vi "Log Into File.vi"(8 "error in":errorcluster, 10 "Memory Information":dbl[](array[numeric]), 11 "file path in":path) -> (0 "error out":errorcluster, 3 "file path out":path)   [LabVIEW 2016]
uses:
  <vilib>/Utility/file.llb/Write Delimited Spreadsheet (string).vi
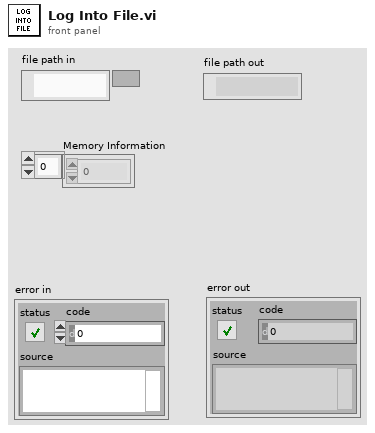
[diagram p1: front panel]
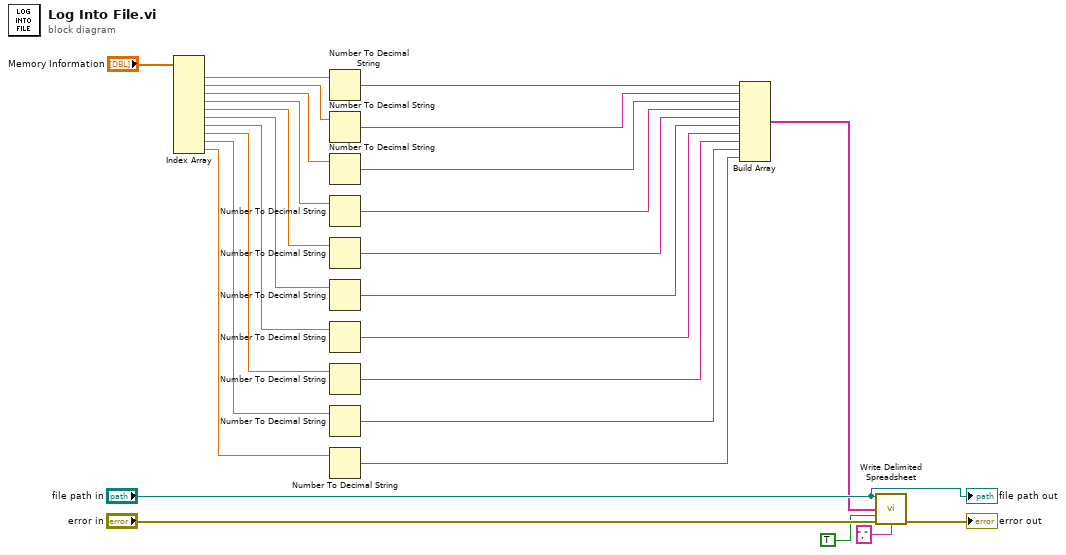
[diagram p0: block diagram]
diagram:
  n1 = Index Array(array="Memory Information") -> (element #1=w26:dbl, element #2=w21:dbl, element #3=w20:dbl, element #4=w19:dbl, element #5=w18:dbl, element #6=w17:dbl, element #7=w16:dbl, element #8=w15:dbl, element #9=w14:dbl, element #10=w13:dbl)  [unwired: 10 in]
  n2 = Number To Decimal String(number=w26) -> (decimal integer string=w11:string)  [unwired: 1 in]
  n3 = Number To Decimal String(number=w21) -> (decimal integer string=w10:string)  [unwired: 1 in]
  n4 = Number To Decimal String(number=w20) -> (decimal integer string=w9:string)  [unwired: 1 in]
  n5 = Number To Decimal String(number=w19) -> (decimal integer string=w8:string)  [unwired: 1 in]
  n6 = Number To Decimal String(number=w18) -> (decimal integer string=w7:string)  [unwired: 1 in]
  n7 = Number To Decimal String(number=w17) -> (decimal integer string=w6:string)  [unwired: 1 in]
  n8 = Number To Decimal String(number=w16) -> (decimal integer string=w5:string)  [unwired: 1 in]
  n9 = Number To Decimal String(number=w15) -> (decimal integer string=w4:string)  [unwired: 1 in]
  n10 = Number To Decimal String(number=w14) -> (decimal integer string=w3:string)  [unwired: 1 in]
  n11 = Number To Decimal String(number=w13) -> (decimal integer string=w2:string)  [unwired: 1 in]
  n12 = Build Array(w11, w10, w9, w8, w7, w6, w5, w4, w3, w2) -> (w1:string[])
  n13 = call-poly <vilib>:"Write Delimited Spreadsheet.vi"("file path (dialog if empty)"="file path in", "1D data"=w1, "append to file? (new file:F)"=TRUE, "error in (no error)"="error in", "delimiter (\\t)"="," ("delimiter (\\t)")) -> ("error out"=→"error out":errorcluster)  [unwired: 9 in, 1 out]
  "file path out" <- "file path in"
